vi "STC31-string-array-to-data.vi"(9 "Starting Index":i32, 11 "Data In (string array)":string[](array[string])) -> (0 "STC31: data output":T1 {"CO2 (ppm)" format="%.2f"}, 2 "STC31: Temp (degC)":dbl format="%.2f", 3 "STC31: CO2 (ppm)":dbl format="%.2f")   [LabVIEW 2021]
uses:
  STC31.ctl
panel:
  out "STC31: Temp":string
  out "STC31: CO2":string
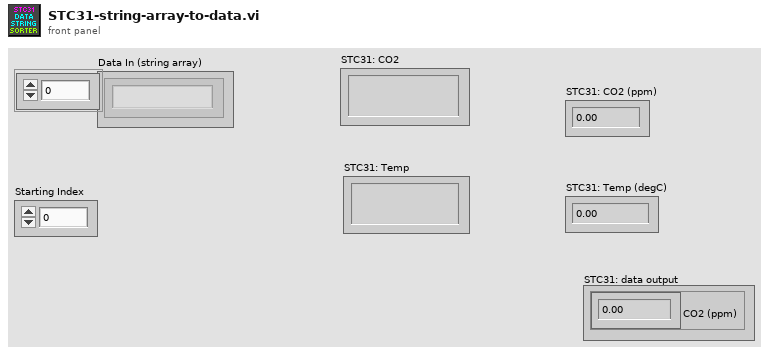
[diagram p1: front panel]
types:
  T1 = typedef "STC31.ctl" = cluster{"CO2 (ppm)":dbl}
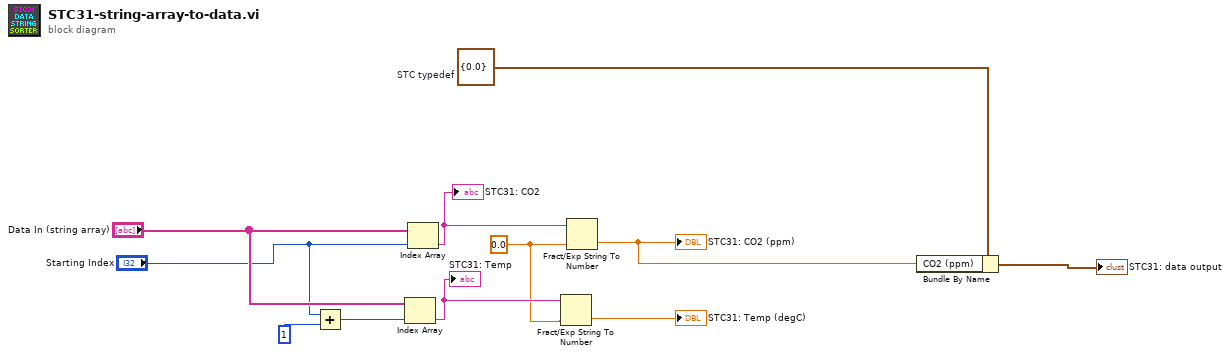
[diagram p0: block diagram]
diagram:
  w3 = T1 {"CO2 (ppm)"=0.0}  # STC typedef
  w5 = 0.0
  n1 = Add(x="Starting Index", y=1) -> (x+y=w9:i32)
  n2 = Index Array(array="Data In (string array)", index=w9) -> (element=w6:string)
  "STC31: Temp" <- w6
  n3 = Index Array "Index Array"(array="Data In (string array)", index="Starting Index") -> (element=w7:string)
  "STC31: CO2" <- w7
  n4 = Fract/Exp String To Number(string=w6, default (0 dbl)=w5) -> (number=→"STC31: Temp (degC)":dbl)  [unwired: 2 in, 1 out]
  n5 = Fract/Exp String To Number(string=w7, default (0 dbl)=w5) -> (number=w2:dbl)  [unwired: 2 in, 1 out]
  "STC31: CO2 (ppm)" <- w2
  n6 = Bundle By Name(cluster=w3, "CO2 (ppm)"=w2) -> (→"STC31: data output":T1)
